vi "ROTPENT_Bal_Control.vi"() -> ()   [LabVIEW 2021]
doc: "This VI is to be used with the NI-ELVIS and the QNET-ROTPENT module. The objective is to learn about balance control of an inverted pendulum, energy control of a pendulum, and a hybrid swing-up controller that integrates the two techniques together."
uses:
  <vilib>/Simulation/Scripting/Companion Diagram/SimConfigNode/SimParams.ctl
  <vilib>/Simulation/Scripting/Companion Diagram/SimConfigNode/_simSolvers.ctl
  <vilib>/Simulation/Implementation/Shared/SIMSCR Execution Mode.ctl
  <vilib>/Platform/TimedLoop/XDataNode/timing_clust.ctl
  <vilib>/Platform/TimedLoop/XDataNode/nitl_modes.ctl
  <vilib>/Platform/TimedLoop/XDataNode/wakeup.ctl
  <vilib>/Simulation/Param Hierarchy/Typedefs/SIMPH Param Control Actions.ctl
  <vilib>/Simulation/Implementation/Shared/NILVSim_ParamChanged.vi
  <vilib>/Simulation/Implementation/Shared/NILVSim_FinishedLate.vi
  <vilib>/Simulation/Implementation/Shared/NILVSIM_BeginStep.vi
  <vilib>/Simulation/DataSources/Implementation/NILVSim Sine Wave.llb/SIM Sine Wave (scalar).vi
  <vilib>/Simulation/Utility/Implementation/SIM Halt.vi
  <vilib>/Simulation/SignalArithmetic/Implementation/NILVSim Gain.llb/SIM Gain (dot product).vi
  <vilib>/Simulation/SignalDisplay/Implementation/NILVSim Time Waveform.llb/SIM Time Waveform (vector).vi
  <vilib>/Simulation/Utility/Implementation/NILVSim Memory.llb/NILVSim Memory (core).vi
  <vilib>/Simulation/SignalDisplay/Implementation/NILVSim Time Waveform.llb/SIM Time Waveform (scalar).vi
  <vilib>/Simulation/Implementation/Shared/NILVSim_Manager.vi
  <vilib>/Utility/error.llb/Clear Errors.vi
  <vilib>/Simulation/Implementation/Shared/NILVSim_FinalizeModel.vi
  <vilib>/Simulation/Implementation/Shared/SIM Unbundle Sim Info.vi
  <vilib>/Simulation/Implementation/Shared/SIMSH Read Queue.vi
  <vilib>/Simulation/Implementation/Shared/NILVSim_Initialize.vi
  QNET Library/conversion_functions/conversion_deg_to_rad.vi
  QNET Library/QNET_Drivers.llb/QNET_ROTPENT_Read_All_Inputs.vi
  <vilib>/Simulation/Utility/Implementation/NILVSim Get Time and IsAcceptedStep.vi
  QNET Library/QNET_ROTPEN_Functions/swingup_pendulum_energy.vi
  QNET Library/QNET_ROTPEN_Functions/QNET_ROTPEN_Enable_Balance.vi
  QNET Library/QNET_ROTPEN_Functions/ROTPENT_Disturbance.vi
  QNET Library/QNET_Drivers.llb/QNET_DCMCT_Motor_Write.vi
  <vilib>/Simulation/Implementation/Shared/NILVSim_GetModelError.vi
  <vilib>/Simulation/Implementation/Shared/SIM Bundle Sim Info.vi
  <vilib>/Simulation/Scripting/Companion Diagram/SimConfigNode/SimDog.xnode
  QNET Library/Simulation_Module_Functions/QNET_Rotpen_Construct_State_Sim - Dera.vi
  <vilib>/Platform/TimedLoop/XDataNode/XDataNode.xnode
  <vilib>/Simulation/Implementation/XNodeFramework/SimXNode/SimX.xnode
  <vilib>/Platform/TimedLoop/XDataNode/XDNodeRunTimeDep.lvlib
  <vilib>/Simulation/Implementation/Shared/NI_SIM_Implementation.lvlib
panel:
  in  "Model Parameters 2":T1={"Mp"=0.027000000700354576, "lp"=0.15299999713897705, "r"=0.08259999752044678, "Jp"=0.000177, "Jeq"=0.00018374, "Kt"=0.0333, "Rm"=8.7, "Bp"=0.0, "Beq"=0.0, "Marm"=0.08} caption="Model Parameters" {"Marm" min=0.0 step=0.0010000000474974513 format="%_3f"; "Beq" min=0 max=0.01 format="%_3g"; "Bp" min=0 max=0.01 format="%_3g"; "Rm" min=0.0 max=10.0 step=0.05000000074505806 format="%_3f"; "Kt" min=0.0 max=0.10000000149011612 step=0.0010000000474974513 format="%_3f"; "Jeq" min=0.0 max=0.0010000000474974513 step=9.999999747378752e-06 format="%_3g"; "Jp" min=0.0 max=0.0010000000474974513 step=9.999999747378752e-06 format="%_3g"; "r" min=0.0 max=0.20000000298023224 step=0.0010000000474974513 format="%_3f"; "lp" min=0.0 max=1.0 step=0.0010000000474974513 format="%#_3f"; "Mp" min=0.0 step=0.0010000000474974513 format="%_3f"}
  in  "theta_reference":dbl=3.141592653589793
  in  "alpha_reference":dbl=3.141592653589793
  in  "Signal Generator 2":cluster{"Signal Type":u16, "Disturbance":bool} caption="Signal Generator"
  in  "Dither Signal":T2={"Amplitude (V)"=0.0, "Frequency (Hz)"=2.5, "Offset (V)"=0.0} {"Offset (V)" min=-2.5 max=2.5 step=0.10000000149011612 format="%_3f"; "Frequency (Hz)" min=0.0 max=50.0 step=0.5 format="%_3f"; "Amplitude (V)" min=0.0 max=5.0 step=0.1 format="%.2f"}
  in  "Balance Control Parameters":T3={"kp_theta (V/rad)"=-6.500000007450581, "kp_alpha (V/rad)"=80.0, "kd_theta (V.s/rad)"=-2.75, "kd_alpha (V.s/rad)"=10.500000022351742} {"kd_alpha (V.s/rad)" min=0.0 max=25.0 step=0.10000000149011612 format="%_3f"; "kd_theta (V.s/rad)" min=-10.0 max=0.0 step=0.10000000149011612 format="%_3f"; "kp_alpha (V/rad)" min=0.0 max=200.0 format="%_3f"; "kp_theta (V/rad)" min=-10.0 max=0.0 step=0.10000000149011612 format="%_3f"}
  out "Digital Scopes":T4={"Current"=-0.3089041535250273, "Voltage"=-0.8694382347063535, "Alpha"=-179.82421875, "Theta"=21.5} {"Theta" format="%.1f"; "Alpha" format="%.1f"; "Voltage" format="%.1f"; "Current" format="%.1f"}
  out "Energy (mJ)":dbl=81.05178567684688 caption="Energy" format="%.1f"
  out "In Range?":bool=TRUE
  in  "Device":tag="Dev1" caption="dev"
  in  "Sampling Rate (Hz)":dbl=100.0 min=0.0 max=1000.0 step=25.0 format="%.1f"
  out "Angle / Energy (deg/mJ)":waveform(dbl)[](graph)=[{"t0"=timestamp(14.780000000000001 s since 1904-01-01), "dt"=1.0, "Y"=[21.5]}, {"t0"=timestamp(14.780000000000001 s since 1904-01-01), "dt"=1.0, "Y"=[-179.82421875]}, {"t0"=timestamp(14.780000000000001 s since 1904-01-01), "dt"=1.0, "Y"=[81.05178567684688]}]
  out "Voltage (V)":waveform(dbl)(graph)={"t0"=timestamp(14.780000000000001 s since 1904-01-01), "dt"=1.0, "Y"=[4.463645732649747]}
  in  "Stop VI":bool caption="CLEAN EXIT"
  # "kg"
  # "m"
  # "kg"
  # "m"
  # "kg.m^2"
  # "kg.m^2"
  # "N.m/A"
  # "ohm"
  # "deg"
  # "deg"
  # "V"
  # "Control Indicators"
  # "mJ"
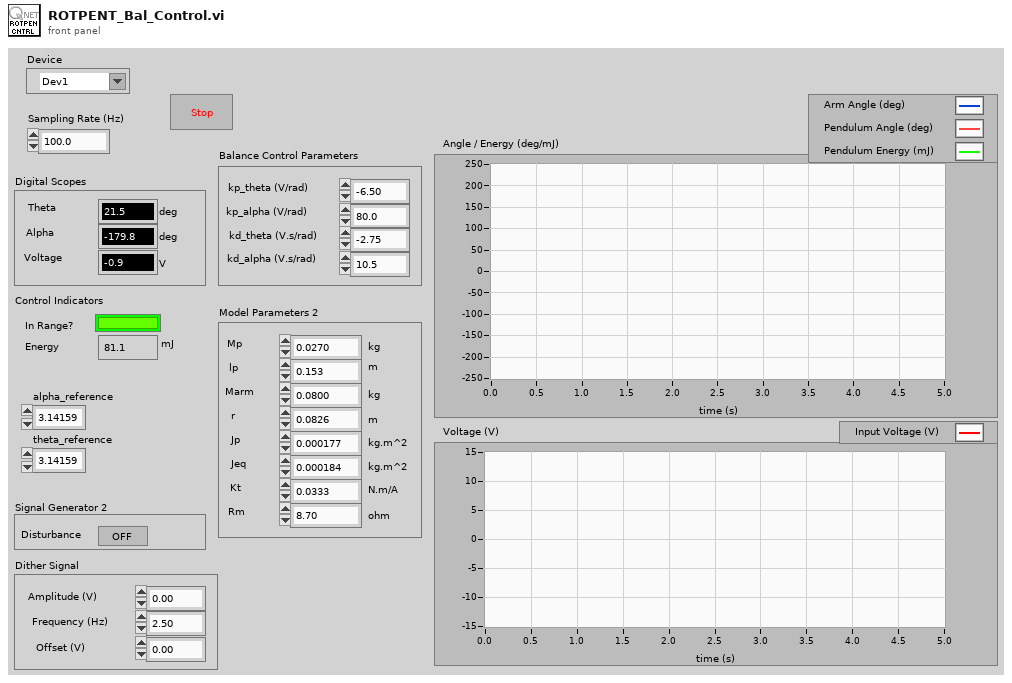
[diagram p1: front panel]
types:
  T1 = cluster{"Mp":dbl, "lp":dbl, "r":dbl, "Jp":dbl, "Jeq":dbl, "Kt":dbl, "Rm":dbl, "Bp":sgl, "Beq":sgl, "Marm":dbl}
  T2 = cluster{"Amplitude (V)":dbl, "Frequency (Hz)":dbl, "Offset (V)":dbl}
  T3 = cluster{"kp_theta (V/rad)":dbl, "kp_alpha (V/rad)":dbl, "kd_theta (V.s/rad)":dbl, "kd_alpha (V.s/rad)":dbl}
  T4 = cluster{"Current":dbl, "Voltage":dbl, "Alpha":dbl, "Theta":dbl}
  T5 = cluster{"link task out":refnum<k21>, "arm task out":refnum<k21>, "spd/curr task out":refnum<k21>}
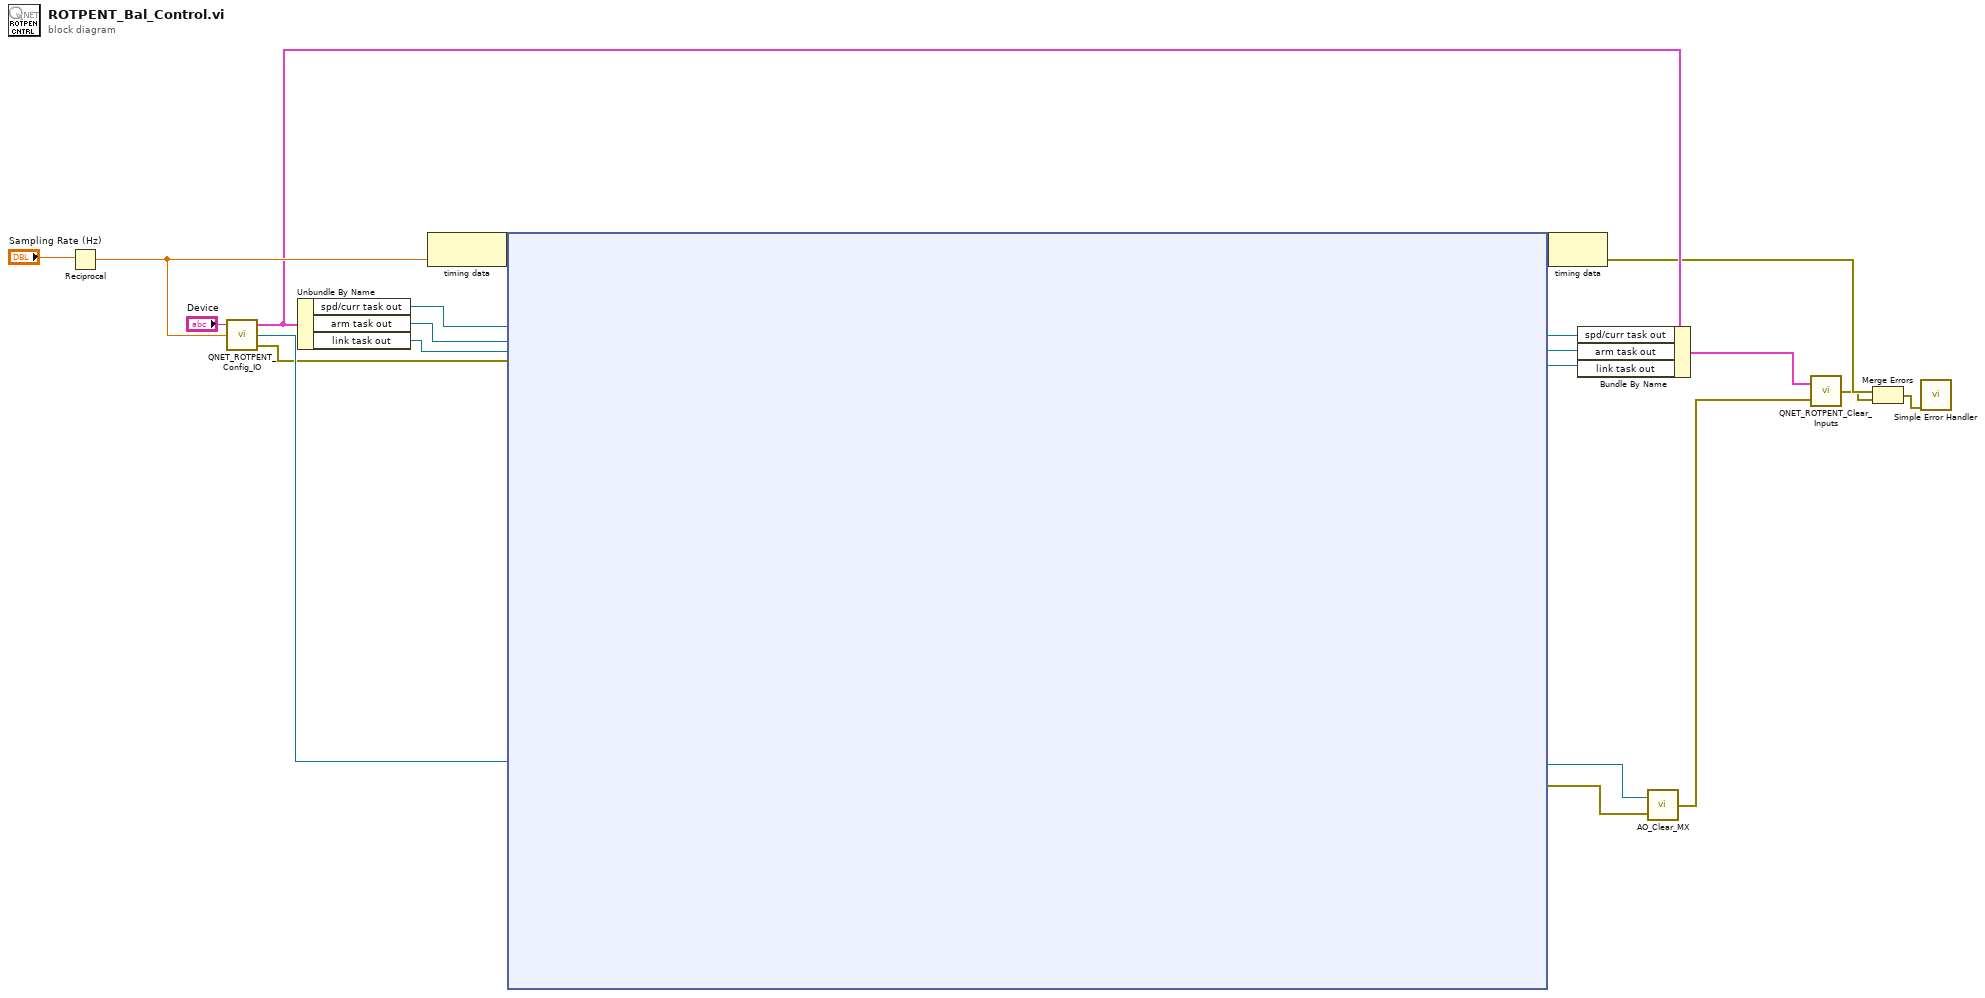
[diagram p0: block diagram]
diagram:
  n1 = Reciprocal(x="Sampling Rate (Hz)") -> (1/x=w9:dbl)
  n2 = call "QNET_ROTPENT_Config_IO.vi"("h (s)"=w9, "dev"="Device") -> ("error out"=w17:errorcluster, "motor task out"=w21:refnum<k21>, "ROTPEN Sensors task out"=w8:T5)  [unwired: 1 in]
  n3 = Unbundle By Name(w8) -> ("spd/curr task out"=w20:refnum<k21>, "arm task out"=w19:refnum<k21>, "link task out"=w18:refnum<k21>)
  n4 = node-c288(w9) -> (w12:variant)
  n5 = node-c254 ("Simulation Loop")(w12, w21, w20, w19, w18, w17) -> (w11:variant, w3:refnum<k21>, w2:refnum<k21>, w1:refnum<k21>, w4:refnum<k21>, w16:errorcluster)
  n6 = node-c288(w11) -> (w7:errorcluster)
  n7 = Bundle By Name(cluster=w8, "spd/curr task out"=w3, "arm task out"=w2, "link task out"=w1) -> (w14:T5)
  n8 = call "AO_Clear_MX.vi"("Error in"=w16, "Task in"=w4) -> ("Error out"=w13:errorcluster)
  n9 = call "QNET_ROTPENT_Clear_Inputs.vi"("Error in"=w13, "ROTPEN Sensors task out"=w14) -> ("Error out"=w6:errorcluster)
  n10 = Merge Errors(w7, w6) -> (w5:errorcluster)
  n11 = call <vilib>:"Simple Error Handler.vi"("error in (no error)"=w5) -> ()  [unwired: 1 in, 8 out]
